vi "Global_ScorePlayer2.vi"() -> ()   [LabVIEW 2018]
panel:
  in  "ScorePlayer2":u16
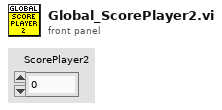
[diagram p1: front panel]
diagram:
